vi "Datafilename.vi"(1 "Position Number":i8, 2 "Rack":u8, 3 "System":u8, 4 "Data File Path":path) -> (0 "File Details":cluster{"Data Path":path, "Position Number":i8})   [LabVIEW 2021]
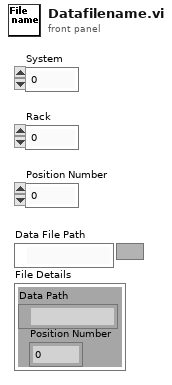
[diagram p1: front panel]
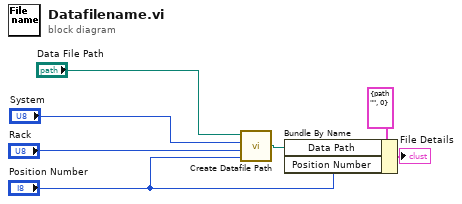
[diagram p0: block diagram]
diagram:
  n1 = call "Create Datafile Path.vi"("Position"="Position Number", "Rack"="Rack", "System"="System", "Data Directory"="Data File Path") -> ("Data Path"=w6:path)
  n2 = Bundle By Name(cluster=cluster{"Data Path":path, "Position Number":i8} {"Data Path"=path "", "Position Number"=0} ("File Details"), "Data Path"=w6, "Position Number"="Position Number") -> (→"File Details":cluster{"Data Path":path, "Position Number":i8})
